vi "FPGA Target 2.vi"() -> ()   [LabVIEW 2015]
uses:
  <vilib>/NI/Engine Simulation Toolkit (EST)/APU/Shared Settings.ctl
  <vilib>/NI/Engine Simulation Toolkit (EST)/Version Token.ctl
  <vilib>/NI/Engine Simulation Toolkit (EST)/APU/Settings.ctl
  <vilib>/NI/Engine Simulation Toolkit (EST)/APU/Input.ctl
  <vilib>/NI/Engine Simulation Toolkit (EST)/APU/Output.ctl
  <vilib>/NI/Engine Simulation Toolkit (EST)/Analog Replay/Load Input.ctl
  <vilib>/NI/FPGA Addon IP/Speciality IO/Types/PWM.Measure.Analog.Settings.ctl
  <vilib>/NI/FPGA Addon IP/Speciality IO/Types/PWM.Measure.Analog.Measurement.ctl
  <vilib>/NI/Engine Simulation Toolkit (EST)/Knock Sensor/Cylinder Settings.ctl
  <vilib>/NI/Engine Simulation Toolkit (EST)/Knock Sensor/Cylinder Input.ctl
  <vilib>/NI/Engine Simulation Toolkit (EST)/Knock Sensor/Generate Settings.ctl
  <vilib>/NI/Engine Simulation Toolkit (EST)/Knock Sensor/Generate Input.ctl
  <vilib>/NI/Engine Simulation Toolkit (EST)/Analog Replay/Input.ctl
  <vilib>/NI/Engine Simulation Toolkit (EST)/Analog Replay/Settings.ctl
  <vilib>/NI/FPGA Addon IP/Speciality IO/Types/Sine.Generate.Settings.ctl
  <vilib>/Platform/TimedLoop/XDataNode/timing_clust.ctl
  <vilib>/Platform/TimedLoop/XDataNode/nitl_modes.ctl
  <vilib>/Platform/TimedLoop/XDataNode/wakeup.ctl
  <vilib>/rvi/Emulation/niFpgaSctlEmulationGetInTimedLoop.vi
  <vilib>/rvi/Emulation/niFpgaEmulationReportErrorSimple.vi
  <vilib>/rvi/Emulation/niFpgaGetClockAttributes.vi
  <vilib>/rvi/Emulation/niFpgaCriticalErrorInLSC.vi
  <vilib>/rvi/Emulation/niFpgaProcessEmulError.vi
  <vilib>/rvi/interface/RandomDataEmulation/niFpgaRandomDataHandleErrors.vi
  <vilib>/Platform/TimedLoop/XDataNode/XDataNode.xnode
  <vilib>/rvi/DataTransferAndStorage/Container/XNode/niFpgaContainer.xnode
  <vilib>/rvi/interface/RandomDataEmulation/nirviRandomDataFpgaReadWriteTemplate.vi
  <vilib>/Platform/TimedLoop/XDataNode/XDNodeRunTimeDep.lvlib
  <vilib>/NI/Engine Simulation Toolkit (EST)/APU/APU.lvlib
  <vilib>/NI/Engine Simulation Toolkit (EST)/Analog Replay/Analog Replay.lvlib
  <vilib>/NI/FPGA Addon IP/Speciality IO/Speciality FPGA IO.lvlib
  <vilib>/NI/Engine Simulation Toolkit (EST)/Knock Sensor/Knock Sensor.lvlib
  <vilib>/NI/Engine Simulation Toolkit (EST)/Engine Simulation Toolkit.lvlib
panel:
  out "Mod2.Monitor":fxp<+/-,32,8>[](array[numeric])
  in  "Simple Knock 2.Settings":T1={"AMP"=0.0, "OFFSET"=0.0, "PERIODS/TICKS"=2.4999957531690598e-05}
  in  "Simple Knock 1.Settings":T1={"AMP"=0.0, "OFFSET"=0.0, "PERIODS/TICKS"=2.4999957531690598e-05}
  in  "input.VR Sensor2":T2
  in  "settings.VR Sensor2":T3
  in  "input.VR Sensor1":T2
  in  "settings.VR Sensor1":T3
  out "Mod1.Monitor":fxp<+/-,32,8>[](array[numeric])
  in  "Power Supply Setpoint":fxp<+/-,32,8> format="%#_27g"
  in  "Dyno Setpoint":fxp<+/-,32,8> format="%#_27g"
  in  "input.Knock2":T4
  in  "settings.Knock2":T5
  in  "input.Knock2.Cylinder 7":T6={"probability compare"=65535, "high freq scaler"=0.0, "trigger position"=0}
  in  "settings.Knock2.Cylinder 7":T7
  in  "input.Knock2.Cylinder 6":T6={"probability compare"=65535, "high freq scaler"=0.0, "trigger position"=0}
  in  "settings.Knock2.Cylinder 6":T7
  in  "input.Knock2.Cylinder 5":T6={"probability compare"=65535, "high freq scaler"=0.0, "trigger position"=0}
  in  "settings.Knock2.Cylinder 5":T7
  in  "input.Knock2.Cylinder 4":T6={"probability compare"=65535, "high freq scaler"=0.0, "trigger position"=0}
  in  "settings.Knock2.Cylinder 4":T7
  in  "input.Knock2.Cylinder 3":T6={"probability compare"=65535, "high freq scaler"=0.0, "trigger position"=0}
  in  "settings.Knock2.Cylinder 3":T7
  in  "input.Knock2.Cylinder 2":T6={"probability compare"=65535, "high freq scaler"=0.0, "trigger position"=0}
  in  "settings.Knock2.Cylinder 2":T7
  in  "input.Knock2.Cylinder 1":T6={"probability compare"=65535, "high freq scaler"=0.0, "trigger position"=0}
  in  "settings.Knock2.Cylinder 1":T7
  in  "input.Knock1":T4
  in  "settings.Knock1":T5
  in  "input.Knock1.Cylinder 6":T6={"probability compare"=65535, "high freq scaler"=0.0, "trigger position"=0}
  in  "settings.Knock1.Cylinder 6":T7
  in  "input.Knock1.Cylinder 5":T6={"probability compare"=65535, "high freq scaler"=0.0, "trigger position"=0}
  in  "settings.Knock1.Cylinder 5":T7
  in  "input.Knock1.Cylinder 4":T6={"probability compare"=65535, "high freq scaler"=0.0, "trigger position"=0}
  in  "settings.Knock1.Cylinder 4":T7
  in  "input.Knock1.Cylinder 3":T6={"probability compare"=65535, "high freq scaler"=0.0, "trigger position"=0}
  in  "settings.Knock1.Cylinder 3":T7
  in  "input.Knock1.Cylinder 2":T6={"probability compare"=65535, "high freq scaler"=0.0, "trigger position"=0}
  in  "settings.Knock1.Cylinder 2":T7
  in  "input.Knock1.Cylinder 1":T6={"probability compare"=65535, "high freq scaler"=0.0, "trigger position"=0}
  in  "settings.Knock1.Cylinder 1":T7
  out "Injector14.Measure":T8
  in  "Injector14.Settings":T9={"ACTIVE EDGE"=TRUE, "TIMEOUT"=40000000, "THRESHOLD"=50.0}
  out "Injector13.Measure":T8
  in  "Injector13.Settings":T9={"ACTIVE EDGE"=TRUE, "TIMEOUT"=40000000, "THRESHOLD"=50.0}
  out "Pressure12":fxp<+/-,32,8> format="%#_27g"
  out "Pressure11":fxp<+/-,32,8> format="%#_27g"
  out "Mod6.Monitor":fxp<+/-,24,5>[](array[numeric])
  out "Injector12.Measure":T8
  in  "Injector12.Settings":T9={"ACTIVE EDGE"=TRUE, "TIMEOUT"=40000000, "THRESHOLD"=50.0}
  out "Injector11.Measure":T8
  in  "Injector11.Settings":T9={"ACTIVE EDGE"=TRUE, "TIMEOUT"=40000000, "THRESHOLD"=50.0}
  out "Pressure10":fxp<+/-,32,8> format="%#_27g"
  out "Pressure9":fxp<+/-,32,8> format="%#_27g"
  out "Mod5.Monitor":fxp<+/-,24,5>[](array[numeric])
  out "Injector10.Measure":T8
  in  "Injector10.Settings":T9={"ACTIVE EDGE"=TRUE, "TIMEOUT"=40000000, "THRESHOLD"=50.0}
  out "Injector9.Measure":T8
  in  "Injector9.Settings":T9={"ACTIVE EDGE"=TRUE, "TIMEOUT"=40000000, "THRESHOLD"=50.0}
  out "Pressure8":fxp<+/-,32,8> format="%#_27g"
  out "Pressure7":fxp<+/-,32,8> format="%#_27g"
  out "Injector8.Measure":T8
  in  "Injector8.Settings":T9={"ACTIVE EDGE"=TRUE, "TIMEOUT"=40000000, "THRESHOLD"=50.0}
  out "Injector7.Measure":T8
  in  "Injector7.Settings":T9={"ACTIVE EDGE"=TRUE, "TIMEOUT"=40000000, "THRESHOLD"=50.0}
  out "Pressure6":fxp<+/-,32,8> format="%#_27g"
  out "Pressure5":fxp<+/-,32,8> format="%#_27g"
  out "Mod4.Monitor":fxp<+/-,16,7>[](array[numeric])
  out "Injector6.Measure":T8
  in  "Injector6.Settings":T9={"ACTIVE EDGE"=TRUE, "TIMEOUT"=40000000, "THRESHOLD"=50.0}
  out "Injector5.Measure":T8
  in  "Injector5.Settings":T9={"ACTIVE EDGE"=TRUE, "TIMEOUT"=40000000, "THRESHOLD"=50.0}
  out "Pressure4":fxp<+/-,32,8> format="%#_27g"
  out "Pressure3":fxp<+/-,32,8> format="%#_27g"
  out "Injector4.Measure":T8
  in  "Injector4.Settings":T9={"ACTIVE EDGE"=TRUE, "TIMEOUT"=40000000, "THRESHOLD"=50.0}
  out "Injector3.Measure":T8
  in  "Injector3.Settings":T9={"ACTIVE EDGE"=TRUE, "TIMEOUT"=40000000, "THRESHOLD"=50.0}
  out "Pressure2":fxp<+/-,32,8> format="%#_27g"
  out "Pressure1":fxp<+/-,32,8> format="%#_27g"
  out "Mod3.Monitor":fxp<+/-,16,5>[](array[numeric])
  in  "load input.VR Sensor2":T10={"Data"=[0, 0, 0, 0, 0, 0, 0, 0, 0, 0, 0, 0, 0, 0, 0, 0], "LoadOffset"=0, "Done"=FALSE}
  in  "load input.VR Sensor1":T10={"Data"=[0, 0, 0, 0, 0, 0, 0, 0, 0, 0, 0, 0, 0, 0, 0, 0], "LoadOffset"=0, "Done"=FALSE}
  out "Actual Analog Input Loop Period (usec)":u32
  out "Actual Analog Output Loop Period (usec)":u32
  out "Actual Digital Loop Period (usec)":u32
  out "Actual DMA Loop Period (usec)":u32
  in  "Analog Input Loop Timer (uSec)":u32
  out "output.apu 1":T11 caption="output"
  in  "input.apu 1":T12={"desired speed"=0.0, "reset"=TRUE} caption="input"
  in  "settings.apu 1":T13 caption="settings"
  in  "est.version":T14
  in  "shared settings.apu 1":T15 {"start" format="%#.15g"}
  in  "go.apu 1":bool
  in  "Digital Loop Timer (uSec)":u32
  in  "Analog Output Loop Timer (uSec)":u32
  in  "DMA.Enable":bool
  in  "DMA.MinimumSamples":u32 caption="DMA Loop Timer (uSec)"
  out "DMA.Timeout":bool
  in  "DMA.Timeout.Reset":bool
  in  "DMA Loop Timer (uSec)":u32
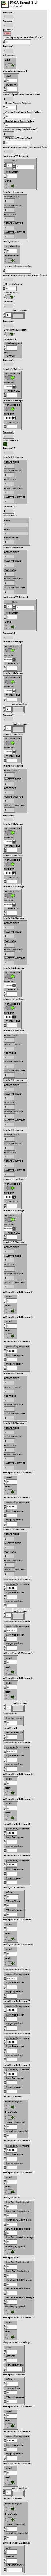
[diagram p1: front panel]
types:
  T1 = typedef "Speciality FPGA IO.lvlib/Sine.Generate.Settings.ctl" = cluster{"AMP":fxp<+/-,32,8>, "OFFSET":fxp<+/-,32,8>, "PERIODS/TICKS":fxp<+,32,0>}
  T2 = typedef "Engine Simulation Toolkit.lvlib/Analog Replay.lvlib/Settings.ctl" = cluster{"ReverseNegate":bool, "CycleAngle":bool, "SpeedThreshold":fxp<+/-,23,2>, "AOBelowThreshold":i16}
  T3 = typedef "Engine Simulation Toolkit.lvlib/Analog Replay.lvlib/Input.ctl" = cluster{"Offset":i16, "VScaleSlope":fxp<+,18,6>, "VScaleIntercept":fxp<+/-,18,3>}
  T4 = typedef "Engine Simulation Toolkit.lvlib/Knock Sensor.lvlib/Generate Input.ctl" = cluster{"low freq scaler":fxp<+,10,0>}
  T5 = typedef "Engine Simulation Toolkit.lvlib/Knock Sensor.lvlib/Generate Settings.ctl" = cluster{"low freq (periods/tick)":fxp<+,32,0>, "high freq (periods/tick)":fxp<+,32,0>, "duration (1.25MHz tics)":fxp<+,18,18>, "low freq speed slope":fxp<+,16,-3>, "low freq speed intercept":fxp<+,10,-10>, "low freq by speed":bool}
  T6 = typedef "Engine Simulation Toolkit.lvlib/Knock Sensor.lvlib/Cylinder Input.ctl" = cluster{"probability compare":u16, "high freq scaler":fxp<+,10,0>, "trigger position":u16}
  T7 = typedef "Engine Simulation Toolkit.lvlib/Knock Sensor.lvlib/Cylinder Settings.ctl" = cluster{"seed":u16, "reset":bool}
  T8 = typedef "Speciality FPGA IO.lvlib/PWM.Measure.Analog.Measurement.ctl" = cluster{"ACTIVE TICKS":u32, "INACTIVE TICKS":u32, "ACQ TICKS":u32, "ACTIVE VOLTAGE":fxp<+/-,32,8>, "INACTIVE VOLTAGE":fxp<+/-,32,8>}
  T9 = typedef "Speciality FPGA IO.lvlib/PWM.Measure.Analog.Settings.ctl" = cluster{"ACTIVE EDGE":bool, "TIMEOUT":u32, "THRESHOLD":fxp<+/-,32,8>}
  T10 = typedef "Engine Simulation Toolkit.lvlib/Analog Replay.lvlib/Load Input.ctl" = cluster{"Data":i16[], "LoadOffset":u16, "Done":bool}
  T11 = typedef "Engine Simulation Toolkit.lvlib/APU.lvlib/Output.ctl" = cluster{"crank":u16, "cycle":u16, "actual speed":fxp<+/-,23,2>}
  T12 = typedef "Engine Simulation Toolkit.lvlib/APU.lvlib/Input.ctl" = cluster{"desired speed":fxp<+/-,23,2>, "reset":bool}
  T13 = typedef "Engine Simulation Toolkit.lvlib/APU.lvlib/Settings.ctl" = cluster{"acceleration":fxp<+,18,-20>, "enable accel":bool}
  T14 = typedef "Engine Simulation Toolkit.lvlib/Version Token.ctl" = cluster{"1.3.0":bool}
  T15 = typedef "Engine Simulation Toolkit.lvlib/APU.lvlib/Shared Settings.ctl" = cluster{"start":fxp<+,17,17>, "stuck limit":fxp<+,18,18>}
  T16 = typedef "XDNodeRunTimeDep.lvlib/timing_clust.ctl" = cluster{"Expected End [f-1]":u64, "Actual End [f-1]":u64, "Finished Late? [f-1]":bool, "Expected End [i-1]":u64, "Actual End [i-1]":u64, "Finished Late? [i-1]":bool, "Expected Start [i]":u64, "Actual Start [i]":u64, "Expected Start [f]":u64, "Actual Start [f]":u64, "Source Name":string, "Structure Name":string, "Period":i64, "Deadline":i64, "Offset":i64, "Start":i64, "Priority":i32, "Timeout":i32, "Mode":T17, "Wakeup Reason":T18, "Error":errorcluster, "Source Type":string, "Secondary Source Type":string, "Global End Time":u64, "Global Start Time":u64, "Frame Duration":u64, "Iteration Duration":u64, "Assigned CPU":i32, "I/O Scan Engine Mode":u32}
  T17 = typedef "XDNodeRunTimeDep.lvlib/nitl_modes.ctl" = enum32{"No Change", "Process missed periods, maintain original phase", "Discard missed periods, maintain original phase", "Process missed periods, ignore original phase", "Discard missed periods, ignore original phase"}
  T18 = typedef "XDNodeRunTimeDep.lvlib/wakeup.ctl" = enum32{"Normal", "Aborted", "Asynchronous wakeup", "Timing source error", "Timed loop error", "Timeout"}
  T19 = cluster{"AO 0":refnum<k21>, "AO 1":refnum<k21>, "AO 2":refnum<k21>, "AO 3":refnum<k21>}
  T20 = cluster{"AI 0":refnum<k21>, "AI 1":refnum<k21>, "AI 2":refnum<k21>, "AI 3":refnum<k21>}
  T21 = cluster{"AI 0":refnum<k21>, "AI 1":refnum<k21>, "AI 2":refnum<k21>, "AI 3":refnum<k21>, "AI 4":refnum<k21>, "AI 5":refnum<k21>, "AI 6":refnum<k21>, "AI 7":refnum<k21>}
  T22 = typedef "Engine Simulation Toolkit.lvlib/APU.lvlib/Register Bus.ctl" = cluster{"Speed":refnum<k21>, "Crank Angle":refnum<k21>, "Cycle Angle":refnum<k21>, "Crank Count":refnum<k21>, "Cycle Count":refnum<k21>, "1.25 MHz Counter":refnum<k21>, "Crank Rollover":refnum<k21>, "Cycle Rollover":refnum<k21>, "shared settings":T15}
  T23 = typedef "Engine Simulation Toolkit.lvlib/Knock Sensor.lvlib/Triggered Cylinder Data.ctl" = cluster{"trigger knock":bool, "high freq scaler":fxp<+,10,0>}
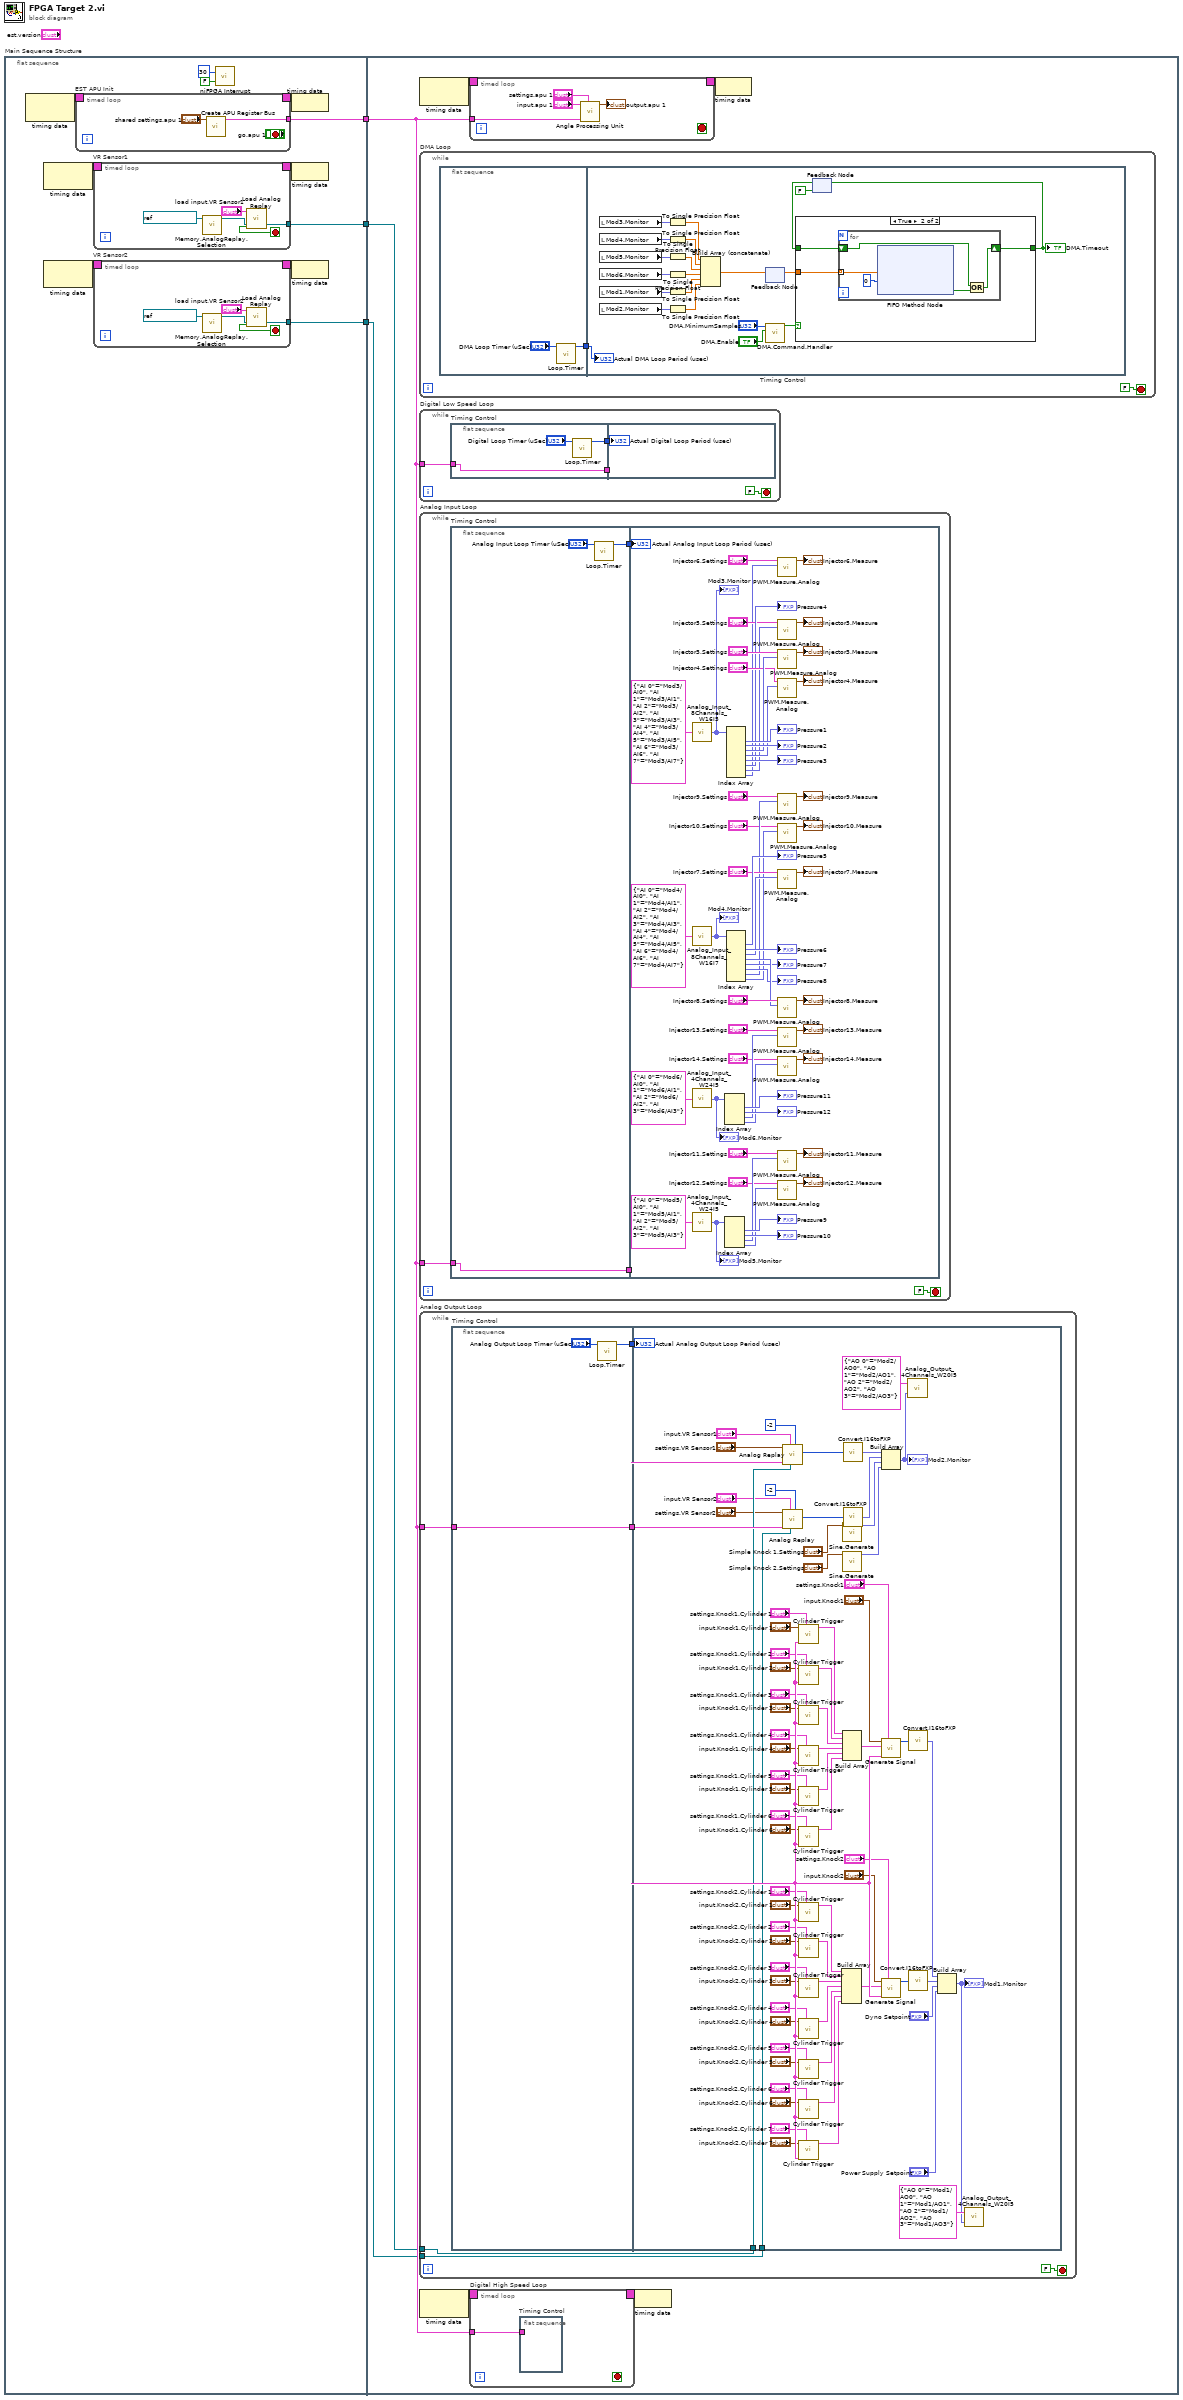
[diagram p0: block diagram]
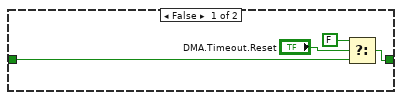
[diagram p2: hidden frame]
diagram:
  n1 = flat-sequence "Main Sequence Structure" {
    tunnel: [w10] -> w3
    tunnel: [w5] -> w2
    tunnel: [w4] -> w1
    tunnel: w3 -> [w40]
    tunnel: w2 -> [w39]
    tunnel: w1 -> [w38]
    frame #0 {
      n2 = node-c288() -> (w12:T16)  [unwired: 1 in]
      n3 = node-c288() -> (w9:T16)  [unwired: 1 in]
      n4 = node-c288() -> (w7:T16)  [unwired: 1 in]
      n5 = timed-loop "EST APU Init" {
        timing: w12 -> [_]
        timing-out: [_] -> w11
        tunnel: [w31] -> w10
        stop <- "go.apu 1" stop-if-true
        n6 = call <vilib>:"Create APU Register Bus.vi"("shared settings.<user name>"="shared settings.apu 1") -> ("register bus"=w31:T22)  [unwired: 10 in]
      }
      n7 = timed-loop "VR Sensor1" {
        timing: w9 -> [_]
        timing-out: [_] -> w8
        tunnel: [w23] -> w5
        stop <- w25 stop-if-true
        n8 = call "Memory.AnalogReplay.Selection.vi"("memory"=refnum<k21> "VR Sensor1") -> ("memory"=w23:refnum<k21>)  [unwired: 10 in]
        n9 = call <vilib>:"Load Analog Replay.vi"("memory"=w23, "load input.<user name>"="load input.VR Sensor1") -> ("done"=w25:bool)  [unwired: 9 in]
      }
      n10 = timed-loop "VR Sensor2" {
        timing: w7 -> [_]
        timing-out: [_] -> w6
        tunnel: [w15] -> w4
        stop <- w17 stop-if-true
        n11 = call "Memory.AnalogReplay.Selection.vi"("memory"=refnum<k21> "VR Sensor2") -> ("memory"=w15:refnum<k21>)  [unwired: 10 in]
        n12 = call <vilib>:"Load Analog Replay.vi"("memory"=w15, "load input.<user name>"="load input.VR Sensor2") -> ("done"=w17:bool)  [unwired: 9 in]
      }
      n13 = call <vilib>:"niFPGA Interrupt.vi"("Wait Until Cleared (F)"=FALSE, "IRQ Number (0)"=u8 30) -> ()  [unwired: 1 in]
      n14 = node-c288(w11) -> ()
      n15 = node-c288(w8) -> ()
      n16 = node-c288(w6) -> ()
    }
    frame #1 {
      # "FPGA Addon Code"
      n17 = node-c288 ("Input Node")() -> (w42:T16)  [unwired: 1 in]
      n18 = while "DMA Loop" {
        stop <- FALSE stop-if-true
        n19 = flat-sequence "Timing Control" {
          tunnel: [w60] -> w58
          tunnel: w58 -> [w74]
          frame #0 {
            n20 = call "Loop.Timer.vi"("Loop Timer (uSec)"="DMA Loop Timer (uSec)") -> ("Actual Loop Period (usec)"=w60:u32)  [unwired: 10 in]
          }
          frame #1 {
            n21 = local read "Mod3.Monitor"() -> (w73:fxp<+/-,16,5>[])
            n22 = local read "Mod4.Monitor"() -> (w72:fxp<+/-,16,7>[])
            n23 = local read "Mod5.Monitor"() -> (w71:fxp<+/-,24,5>[])
            n24 = local read "Mod6.Monitor"() -> (w70:fxp<+/-,24,5>[])
            n25 = local read "Mod1.Monitor"() -> (w69:fxp<+/-,32,8>[])
            n26 = local read "Mod2.Monitor"() -> (w68:fxp<+/-,32,8>[])
            n27 = To Single Precision Float(number=w73) -> (single precision float=w67:sgl[])
            n28 = To Single Precision Float(number=w72) -> (single precision float=w66:sgl[])
            n29 = To Single Precision Float(number=w71) -> (single precision float=w65:sgl[])
            n30 = To Single Precision Float(number=w70) -> (single precision float=w64:sgl[])
            n31 = To Single Precision Float(number=w69) -> (single precision float=w63:sgl[])
            n32 = To Single Precision Float(number=w68) -> (single precision float=w62:sgl[])
            n33 = Build Array (concatenate) "Build Array"(w67, w66, w65, w64, w63, w62) -> (w80:sgl[])
            n34 = feedback #1() -> (w79:sgl[])  [unwired: 1 in]
            n35 = feedback-in #1(w80) -> ()
            n36 = call "DMA.Command.Handler.vi"("DMA.Enable"="DMA.Enable", "DMA.MinimumSamples"="DMA.MinimumSamples") -> ("Transfer"=w76:bool)  [unwired: 9 in]
            n37 = feedback #2(FALSE ("t")) -> (w75:bool)
            n38 = case shown="True" w76 {
              tunnel: w79 -> [_ w89]
              tunnel: w75 -> [w84 w88]
              tunnel: [w83 w87] -> w78
              frame False {
                n39 = Select(t=FALSE, s="DMA.Timeout.Reset", f=w84) -> (s? t:f=w83:bool)
              }
              frame True {
                n40 = for {
                  shift-right: [w92] -> w87
                  shift-left: w88 -> [w91]
                  tunnel: w89 -> [w90] mode=indexing
                  n41 = xnode ("FIFO Method Node")("Element"=w90, "Timeout"=0) -> ("Timed Out?"=w93:bool)  [unwired: 1 in, 1 out]
                  n42 = Or(x=w91, y=w93) -> (x .or. y?=w92:bool)
                }
              }
            }
            "DMA.Timeout" <- w78
            n43 = feedback-in #2(w78) -> ()
            "Actual DMA Loop Period (usec)" <- w74
          }
        }
      }
      n44 = while "Digital Low Speed Loop" {
        tunnel: w40 -> [w243]
        stop <- FALSE stop-if-true
        n45 = flat-sequence "Timing Control" {
          tunnel: w243 -> [w247]
          tunnel: [w247] -> w242
          tunnel: [w245] -> w241
          tunnel: w242 -> [_]
          tunnel: w241 -> [w248]
          frame #0 {
            n46 = call "Loop.Timer.vi"("Loop Timer (uSec)"="Digital Loop Timer (uSec)") -> ("Actual Loop Period (usec)"=w245:u32)  [unwired: 10 in]
          }
          frame #1 {
            "Actual Digital Loop Period (usec)" <- w248
          }
        }
      }
      n47 = while "Analog Input Loop" {
        tunnel: w40 -> [w179]
        stop <- FALSE stop-if-true
        n48 = flat-sequence "Timing Control" {
          tunnel: w179 -> [w183]
          tunnel: [w183] -> w178
          tunnel: [w181] -> w177
          tunnel: w178 -> [_]
          tunnel: w177 -> [w240]
          frame #0 {
            n49 = call "Loop.Timer.vi"("Loop Timer (uSec)"="Analog Input Loop Timer (uSec)") -> ("Actual Loop Period (usec)"=w181:u32)  [unwired: 10 in]
          }
          frame #1 {
            n50 = call "Analog_Input_8Channels_W16I5.vi"("IO"=T21 {"AI 0"="Mod3/AI0", "AI 1"="Mod3/AI1", "AI 2"="Mod3/AI2", "AI 3"="Mod3/AI3", "AI 4"="Mod3/AI4", "AI 5"="Mod3/AI5", "AI 6"="Mod3/AI6", "AI 7"="Mod3/AI7"}) -> ("Values"=w238:fxp<+/-,16,5>[])
            "Mod3.Monitor" <- w238
            n51 = call "Analog_Input_8Channels_W16I7.vi"("IO"=T21 {"AI 0"="Mod4/AI0", "AI 1"="Mod4/AI1", "AI 2"="Mod4/AI2", "AI 3"="Mod4/AI3", "AI 4"="Mod4/AI4", "AI 5"="Mod4/AI5", "AI 6"="Mod4/AI6", "AI 7"="Mod4/AI7"}) -> ("Values"=w220:fxp<+/-,16,7>[])
            "Mod4.Monitor" <- w220
            n52 = call "Analog_Input_4Channels_W24I5.vi"("IO"=T20 {"AI 0"="Mod6/AI0", "AI 1"="Mod6/AI1", "AI 2"="Mod6/AI2", "AI 3"="Mod6/AI3"}) -> ("Values"=w192:fxp<+/-,24,5>[])
            "Mod6.Monitor" <- w192
            n53 = call "Analog_Input_4Channels_W24I5.vi"("IO"=T20 {"AI 0"="Mod5/AI0", "AI 1"="Mod5/AI1", "AI 2"="Mod5/AI2", "AI 3"="Mod5/AI3"}) -> ("Values"=w202:fxp<+/-,24,5>[])
            "Mod5.Monitor" <- w202
            n54 = Index Array(array=w192) -> (element #1=→"Pressure11":fxp<+/-,24,5>, element #2=→"Pressure12":fxp<+/-,24,5>, element #3=w188:fxp<+/-,24,5>, element #4=w185:fxp<+/-,24,5>)  [unwired: 4 in]
            n55 = Index Array(array=w202) -> (element #1=→"Pressure9":fxp<+/-,24,5>, element #2=→"Pressure10":fxp<+/-,24,5>, element #3=w198:fxp<+/-,24,5>, element #4=w195:fxp<+/-,24,5>)  [unwired: 4 in]
            n56 = Index Array(array=w238) -> (element #1=→"Pressure1":fxp<+/-,16,5>, element #2=→"Pressure2":fxp<+/-,16,5>, element #3=w234:fxp<+/-,16,5>, element #4=w231:fxp<+/-,16,5>, element #5=→"Pressure3":fxp<+/-,16,5>, element #6=→"Pressure4":fxp<+/-,16,5>, element #7=w226:fxp<+/-,16,5>, element #8=w223:fxp<+/-,16,5>)  [unwired: 8 in]
            n57 = Index Array(array=w220) -> (element #1=→"Pressure5":fxp<+/-,16,7>, element #2=→"Pressure6":fxp<+/-,16,7>, element #3=w216:fxp<+/-,16,7>, element #4=w213:fxp<+/-,16,7>, element #5=→"Pressure7":fxp<+/-,16,7>, element #6=→"Pressure8":fxp<+/-,16,7>, element #7=w208:fxp<+/-,16,7>, element #8=w205:fxp<+/-,16,7>)  [unwired: 8 in]
            n58 = call <vilib>:"PWM.Measure.Analog.vi"("PWM"=w223, "Settings"="Injector6.Settings") -> ("Measurement"=→"Injector6.Measure":T8)  [unwired: 8 in, 1 out]
            n59 = call <vilib>:"PWM.Measure.Analog.vi"("PWM"=w226, "Settings"="Injector5.Settings") -> ("Measurement"=→"Injector5.Measure":T8)  [unwired: 8 in, 1 out]
            n60 = call <vilib>:"PWM.Measure.Analog.vi"("PWM"=w234, "Settings"="Injector3.Settings") -> ("Measurement"=→"Injector3.Measure":T8)  [unwired: 8 in, 1 out]
            n61 = call <vilib>:"PWM.Measure.Analog.vi"("PWM"=w231, "Settings"="Injector4.Settings") -> ("Measurement"=→"Injector4.Measure":T8)  [unwired: 8 in, 1 out]
            n62 = call <vilib>:"PWM.Measure.Analog.vi"("PWM"=w208, "Settings"="Injector9.Settings") -> ("Measurement"=→"Injector9.Measure":T8)  [unwired: 8 in, 1 out]
            n63 = call <vilib>:"PWM.Measure.Analog.vi"("PWM"=w205, "Settings"="Injector10.Settings") -> ("Measurement"=→"Injector10.Measure":T8)  [unwired: 8 in, 1 out]
            n64 = call <vilib>:"PWM.Measure.Analog.vi"("PWM"=w216, "Settings"="Injector7.Settings") -> ("Measurement"=→"Injector7.Measure":T8)  [unwired: 8 in, 1 out]
            n65 = call <vilib>:"PWM.Measure.Analog.vi"("PWM"=w213, "Settings"="Injector8.Settings") -> ("Measurement"=→"Injector8.Measure":T8)  [unwired: 8 in, 1 out]
            n66 = call <vilib>:"PWM.Measure.Analog.vi"("PWM"=w188, "Settings"="Injector13.Settings") -> ("Measurement"=→"Injector13.Measure":T8)  [unwired: 8 in, 1 out]
            n67 = call <vilib>:"PWM.Measure.Analog.vi"("PWM"=w185, "Settings"="Injector14.Settings") -> ("Measurement"=→"Injector14.Measure":T8)  [unwired: 8 in, 1 out]
            n68 = call <vilib>:"PWM.Measure.Analog.vi"("PWM"=w198, "Settings"="Injector11.Settings") -> ("Measurement"=→"Injector11.Measure":T8)  [unwired: 8 in, 1 out]
            n69 = call <vilib>:"PWM.Measure.Analog.vi"("PWM"=w195, "Settings"="Injector12.Settings") -> ("Measurement"=→"Injector12.Measure":T8)  [unwired: 8 in, 1 out]
            "Actual Analog Input Loop Period (usec)" <- w240
          }
        }
      }
      n70 = while "Analog Output Loop" {
        tunnel: w40 -> [w99]
        tunnel: w39 -> [w96]
        tunnel: w38 -> [w95]
        stop <- FALSE stop-if-true
        n71 = flat-sequence "Timing Control" {
          tunnel: w99 -> [w103]
          tunnel: [w103] -> w98
          tunnel: [w101] -> w97
          tunnel: w98 -> [w173]
          tunnel: w97 -> [w176]
          tunnel: w96 -> [w118]
          tunnel: w95 -> [w113]
          frame #0 {
            n72 = call "Loop.Timer.vi"("Loop Timer (uSec)"="Analog Output Loop Timer (uSec)") -> ("Actual Loop Period (usec)"=w101:u32)  [unwired: 10 in]
          }
          frame #1 {
            n73 = call <vilib>:"Analog Replay.vi"("shift"=i8 -2, "memory"=w118, "settings.<user name>"="input.VR Sensor1", "register bus"=w173, "input.<user name>"="settings.VR Sensor1") -> ("analog value"=w117:i16)  [unwired: 6 in]
            n74 = call <vilib>:"Analog Replay.vi"("shift"=i8 -2, "memory"=w113, "settings.<user name>"="input.VR Sensor2", "register bus"=w173, "input.<user name>"="settings.VR Sensor2") -> ("analog value"=w112:i16)  [unwired: 6 in]
            n75 = call <vilib>:"Cylinder Trigger.vi"("settings.<user name>"="settings.Knock1.Cylinder 1", "register bus"=w173, "input.<user name>"="input.Knock1.Cylinder 1") -> ("triggered knock data"=w172:T23)  [unwired: 8 in]
            n76 = call <vilib>:"Cylinder Trigger.vi"("settings.<user name>"="settings.Knock1.Cylinder 2", "register bus"=w173, "input.<user name>"="input.Knock1.Cylinder 2") -> ("triggered knock data"=w169:T23)  [unwired: 8 in]
            n77 = call <vilib>:"Cylinder Trigger.vi"("settings.<user name>"="settings.Knock1.Cylinder 3", "register bus"=w173, "input.<user name>"="input.Knock1.Cylinder 3") -> ("triggered knock data"=w166:T23)  [unwired: 8 in]
            n78 = call <vilib>:"Cylinder Trigger.vi"("settings.<user name>"="settings.Knock1.Cylinder 4", "register bus"=w173, "input.<user name>"="input.Knock1.Cylinder 4") -> ("triggered knock data"=w163:T23)  [unwired: 8 in]
            n79 = call <vilib>:"Cylinder Trigger.vi"("settings.<user name>"="settings.Knock1.Cylinder 5", "register bus"=w173, "input.<user name>"="input.Knock1.Cylinder 5") -> ("triggered knock data"=w160:T23)  [unwired: 8 in]
            n80 = call <vilib>:"Cylinder Trigger.vi"("settings.<user name>"="settings.Knock1.Cylinder 6", "register bus"=w173, "input.<user name>"="input.Knock1.Cylinder 6") -> ("triggered knock data"=w157:T23)  [unwired: 8 in]
            n81 = call <vilib>:"Cylinder Trigger.vi"("settings.<user name>"="settings.Knock2.Cylinder 1", "register bus"=w173, "input.<user name>"="input.Knock2.Cylinder 1") -> ("triggered knock data"=w150:T23)  [unwired: 8 in]
            n82 = call <vilib>:"Cylinder Trigger.vi"("settings.<user name>"="settings.Knock2.Cylinder 2", "register bus"=w173, "input.<user name>"="input.Knock2.Cylinder 2") -> ("triggered knock data"=w147:T23)  [unwired: 8 in]
            n83 = call <vilib>:"Cylinder Trigger.vi"("settings.<user name>"="settings.Knock2.Cylinder 3", "register bus"=w173, "input.<user name>"="input.Knock2.Cylinder 3") -> ("triggered knock data"=w144:T23)  [unwired: 8 in]
            n84 = call <vilib>:"Cylinder Trigger.vi"("settings.<user name>"="settings.Knock2.Cylinder 4", "register bus"=w173, "input.<user name>"="input.Knock2.Cylinder 4") -> ("triggered knock data"=w141:T23)  [unwired: 8 in]
            n85 = call <vilib>:"Cylinder Trigger.vi"("settings.<user name>"="settings.Knock2.Cylinder 5", "register bus"=w173, "input.<user name>"="input.Knock2.Cylinder 5") -> ("triggered knock data"=w138:T23)  [unwired: 8 in]
            n86 = call <vilib>:"Cylinder Trigger.vi"("settings.<user name>"="settings.Knock2.Cylinder 6", "register bus"=w173, "input.<user name>"="input.Knock2.Cylinder 6") -> ("triggered knock data"=w135:T23)  [unwired: 8 in]
            n87 = call <vilib>:"Cylinder Trigger.vi"("settings.<user name>"="settings.Knock2.Cylinder 7", "register bus"=w173, "input.<user name>"="input.Knock2.Cylinder 7") -> ("triggered knock data"=w132:T23)  [unwired: 8 in]
            n88 = Build Array(w150, w147, w144, w141, w138, w135, w132) -> (w129:T23[])
            n89 = call <vilib>:"Sine.Generate.vi"("Settings"="Simple Knock 1.Settings") -> ("Output"=w107:fxp<+/-,32,8>)  [unwired: 10 in]
            n90 = call <vilib>:"Sine.Generate.vi"("Settings"="Simple Knock 2.Settings") -> ("Output"=w106:fxp<+/-,32,8>)  [unwired: 10 in]
            n91 = Build Array(w172, w169, w166, w163, w160, w157) -> (w154:T23[])
            n92 = call "Convert.I16toFXP.vi"("16bit integer"=w117) -> ("x*y"=w109:fxp<+/-,20,5>)  [unwired: 4 in]
            n93 = call "Convert.I16toFXP.vi"("16bit integer"=w112) -> ("x*y"=w108:fxp<+/-,20,5>)  [unwired: 4 in]
            n94 = Build Array(w109, w108, w107, w106) -> (w104:fxp<+/-,32,8>[])
            "Mod2.Monitor" <- w104
            n95 = call <vilib>:"Generate Signal.vi"("settings.<user name>"="settings.Knock1", "register bus"=w173, "triggered knock data"=w154, "input.<user name>"="input.Knock1") -> ("knock signal"=w153:i16)  [unwired: 7 in]
            n96 = call <vilib>:"Generate Signal.vi"("settings.<user name>"="settings.Knock2", "register bus"=w173, "triggered knock data"=w129, "input.<user name>"="input.Knock2") -> ("knock signal"=w128:i16)  [unwired: 7 in]
            n97 = call "Analog_Output_4Channels_W20I5.vi"("Values"=w104, "IO"=T19 {"AO 0"="Mod2/AO0", "AO 1"="Mod2/AO1", "AO 2"="Mod2/AO2", "AO 3"="Mod2/AO3"}) -> ()  [unwired: 1 in]
            n98 = call "Convert.I16toFXP.vi"("16bit integer"=w153) -> ("x*y"=w127:fxp<+/-,20,5>)  [unwired: 4 in]
            n99 = call "Convert.I16toFXP.vi"("16bit integer"=w128) -> ("x*y"=w126:fxp<+/-,20,5>)  [unwired: 4 in]
            n100 = Build Array(w127, w126, "Dyno Setpoint", "Power Supply Setpoint") -> (w122:fxp<+/-,32,8>[])
            "Mod1.Monitor" <- w122
            n101 = call "Analog_Output_4Channels_W20I5.vi"("Values"=w122, "IO"=T19 {"AO 0"="Mod1/AO0", "AO 1"="Mod1/AO1", "AO 2"="Mod1/AO2", "AO 3"="Mod1/AO3"}) -> ()  [unwired: 1 in]
            "Actual Analog Output Loop Period (usec)" <- w176
          }
        }
      }
      n102 = node-c288() -> (w44:T16)  [unwired: 1 in]
      n103 = timed-loop "Timed Loop" {
        timing: w42 -> [_]
        timing-out: [_] -> w41
        tunnel: w40 -> [w45]
        stop <- _ stop-if-true
        n104 = call <vilib>:"Angle Processing Unit.vi"("settings.<user name>"="settings.apu 1", "register bus"=w45, "input.<user name>"="input.apu 1") -> ("output.<user name>"=→"output.apu 1":T11)  [unwired: 8 in]
      }
      n105 = timed-loop "Digital High Speed Loop" {
        timing: w44 -> [_]
        timing-out: [_] -> w43
        tunnel: w40 -> [w53]
        stop <- _ stop-if-true
        n106 = flat-sequence "Timing Control" {
          tunnel: w53 -> [_]
          frame #0 {
          }
        }
      }
      n107 = node-c288 ("Output Node")(w43) -> ()
      n108 = node-c288 ("Output Node")(w41) -> ()
    }
  }
